vi "Convert to InHg.vi"(11 "Raw V":dbl) -> (2 "Pressure(psi)":dbl, 3 "Vacuum(psi)":dbl)   [LabVIEW 2020]
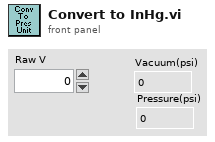
[diagram p1: front panel]
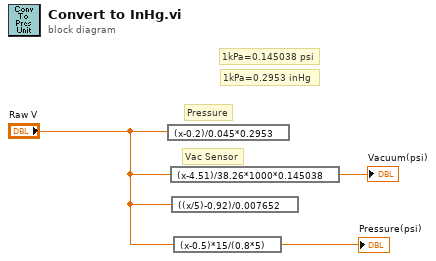
[diagram p0: block diagram]
diagram:
  # "1kPa=0.145038 psi"
  # "Vac Sensor"
  # "Pressure"
  # "1kPa=0.2953 inHg"
  n1 = expression code="(x-0.2)/0.045*0.2953"("Raw V") -> ()  [unwired: 1 out]
  n2 = expression code="(x-4.51)/38.26*1000*0.145038"("Raw V") -> (→"Vacuum(psi)":dbl)
  n3 = expression code="((x/5)-0.92)/0.007652"("Raw V") -> ()  [unwired: 1 out]
  n4 = expression code="(x-0.5)*15/(0.8*5)"("Raw V") -> (→"Pressure(psi)":dbl)
